vi "GetVISAResourceName.vi"(8 "error in (no error)":errorcluster, 11 "object in":refnum<class "PowerSupply.lvclass">) -> (0 "error out":errorcluster, 2 "VISA resource name":refnum<visa-resource-name>, 3 "object out":refnum<class "PowerSupply.lvclass">)   [LabVIEW 2023, in "HardwareAbstractionLayer_LVOOP.lvlib" / "PowerSupply.lvclass"]
uses:
  PowerSupply.lvclass
  PowerSupply.lvclass/PowerSupply.ctl
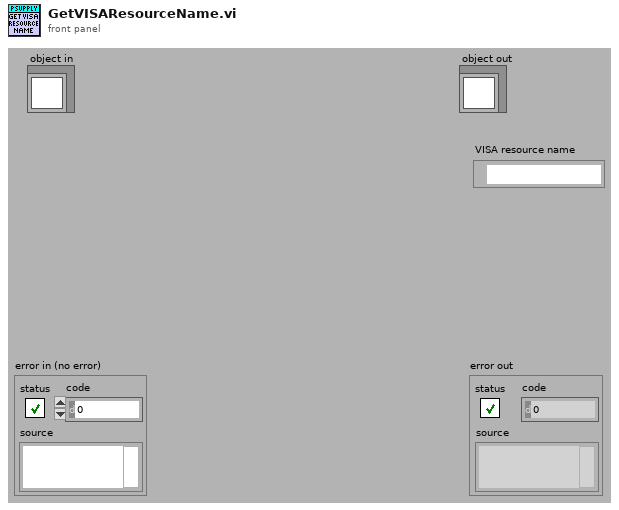
[diagram p1: front panel]
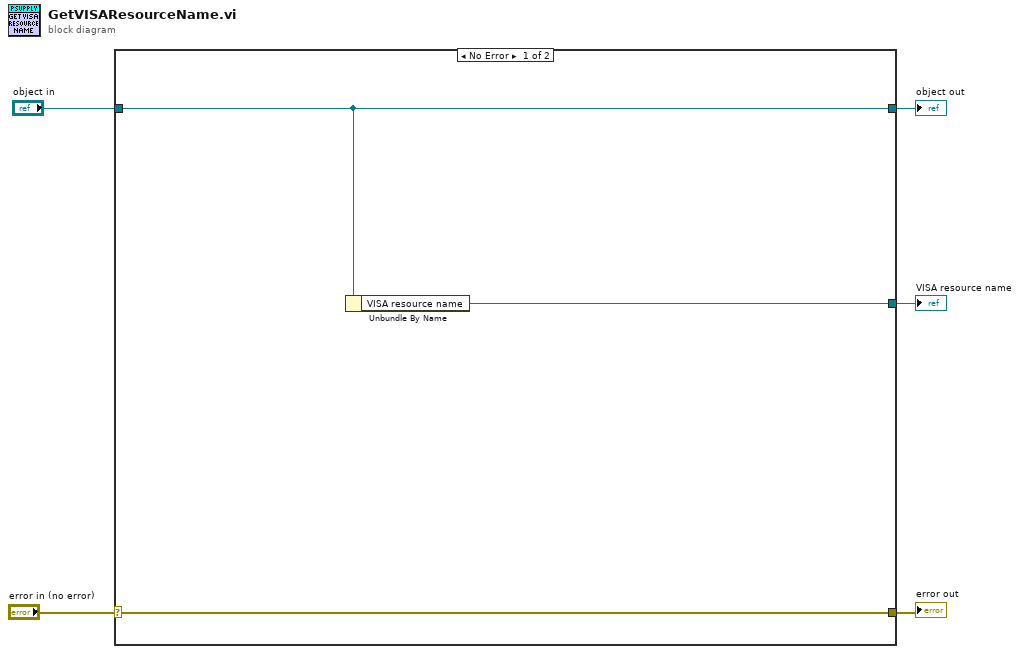
[diagram p0: block diagram]
diagram:
  n1 = case shown="No Error" "error in (no error)" {
    selector: "error in (no error)" -> [w7 w10]
    tunnel: [w7 w10] -> w4
    tunnel: [w6 w9] -> w2
    tunnel: "object in" -> [w6 w9]
    tunnel: [w8 _] -> w1
    frame No Error {
      n2 = Unbundle By Name(w6) -> ("VISA resource name"=w8:refnum<visa-resource-name>)
    }
    frame Error {
    }
  }
  "error out" <- w4
  "object out" <- w2
  "VISA resource name" <- w1
